vi "M05 Solar Cells.vi"(11 "EV3 in":T1) -> ()   [LabVIEW 2016]
uses:
  <vilib>/NXT/Subs/LVHSConnector.ctl
  <vilib>/NXT/LegoClasses/BrickReference/BrickReference.lvclass
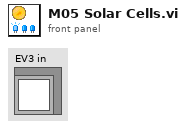
[diagram p1: front panel]
types:
  T1 = typedef "LVHSConnector.ctl" = refnum<class "BrickReference.lvclass">
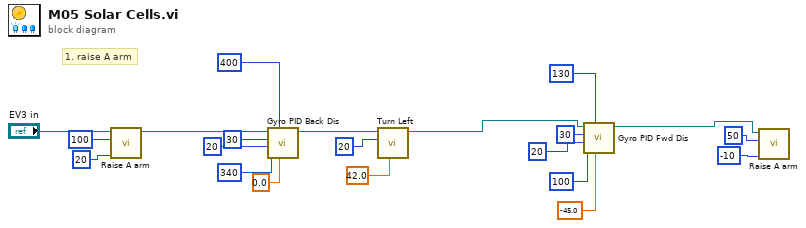
[diagram p0: block diagram]
diagram:
  # "1. raise A arm"
  n1 = call "Raise A arm.vi"("Power"=i8 20, "Rotation"=100, "EV3 in"="EV3 in") -> ("EV3 out"=w18:T1)  [unwired: 8 in]
  n2 = call "Gyro PID Back Dis.vi"("Target angle"=sgl 0.0, "Threshold to stop"=400 ("Threshold to Color"), "Threshold to slow"=340, "Min. speed"=20, "Max. speed"=30, "EV3 in"=w18) -> ("EV3 out"=w12:T1)  [unwired: 5 in]
  n3 = call "Turn Left.vi"("Turning angle"=sgl 42.0, "Motor B (right)"=i8 20, "EV3 in"=w12) -> ("EV3 out"=w2:T1)  [unwired: 8 in]
  n4 = call "Gyro PID Fwd Dis.vi"("Target angle"=sgl -45.0, "Threshold to stop"=130, "Threshold to slow"=100, "Min. speed"=20, "Max. speed"=30, "EV3 in"=w2) -> ("EV3 out"=w1:T1)  [unwired: 5 in]
  n5 = call "Raise A arm.vi"("Power"=i8 -10, "Rotation"=50, "EV3 in"=w1) -> ()  [unwired: 8 in, 1 out]
